vi "Returning A Value Pointer To Complex Struct Added.vi"(8 "error in (no error)":errorcluster) -> (0 "error out":errorcluster, 3 "function return":i64)   [LabVIEW 2009, in "LabVIEWWrapper_PassingDataSampleDLL.lvlib"]
doc: "int ReturningAValue_Integer (void);"
uses:
  LabVIEWWrapper_PassingDataSampleDLL.lvlib
  CustomControlsForStructs/ComplexStruct Polygon.ctl
  PassingDataSampleDLL.dll
panel:
  out "ComplexStruct Polygon":T1
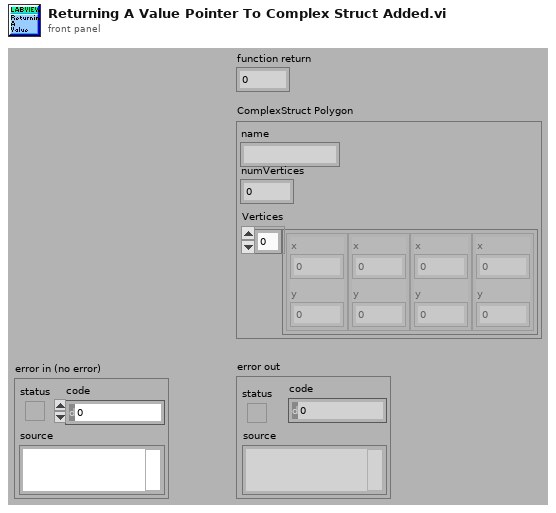
[diagram p1: front panel]
types:
  T1 = typedef "LabVIEWWrapper_PassingDataSampleDLL.lvlib/ComplexStruct Polygon.ctl" = cluster{"name":string, "numVertices":i32, "Vertices":cluster{"x":i32, "y":i32}[]}
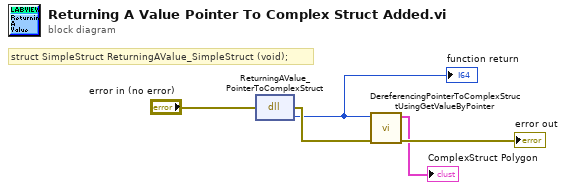
[diagram p0: block diagram]
diagram:
  # "struct SimpleStruct ReturningAValue_SimpleStruct (void);"
  n1 = dll-call lib="C:/My Dropbox/Systems Engineering Application/SDK/C Integration/LabVIEWWrapper/PassingDataSampleDLL.*" fn="ReturningAValue_PointerToComplexStruct"(error in="error in (no error)") -> (error out=w2:errorcluster, "return type"=w1:i64)  [unwired: 2 in, 1 out]
  "function return" <- w1
  n2 = call "DereferencingPointerToComplexStructUsingGetValueByPointer.vi"("error in (no error)"=w2, "Pointer"=w1) -> ("error out"=→"error out":errorcluster, "ComplexStruct Polygon"=→"ComplexStruct Polygon":T1)  [unwired: 8 in]
